vi "Execute.vi"(8 "error in (no error)":errorcluster, 10 "Shifted Error in":refnum<class "Error.lvclass">, 11 "ERROR_Write in":refnum<class "ERROR_Write.lvclass">) -> (0 "error out":errorcluster, 1 "STOP?":bool, 2 "Shifted Error out":refnum<class "Error.lvclass">, 3 "ERROR_Write out":refnum<class "ERROR_Write.lvclass">)   [LabVIEW 2019, in "TSC Error.lvlib" / "ERROR_Write.lvclass"]
doc: "This VI will write the error information to an error log. It contains the following data:\n\nDate String Time String\nVI Name\nMessage: \nGenerated Error Message\n\nInputs:\n-ERROR_Write in [obj] - the dynamic dispatch input class\n-Shifted Error in [obj] - the shifted error class with shared information\n-error in\n\nOutputs:\n-ERROR_Write out [obj] - the dynamic dispatch output class\n-Shifted Error in [obj] - the shifted error class with shared information\n-STOP? [Boolean] - the output Boolean used to stop the Error Loop\n-error out\n\n<b>Code Developed By:</b>\nDaniel Coons\nTechnology Service Corporation\n1983 S Liberty Drive\nBloomington, IN 47403\nPhone: 812 558-7100\nwww.tsc.com/atcs"
uses:
  ERROR_Write.lvclass
  C:/Development/Open Source/tsc-error-library/_Messages/Error/Error.lvclass
  Error/Error.lvclass
  <vilib>/Utility/error.llb/DialogType.ctl
  Error/Error.lvclass/Error.ctl
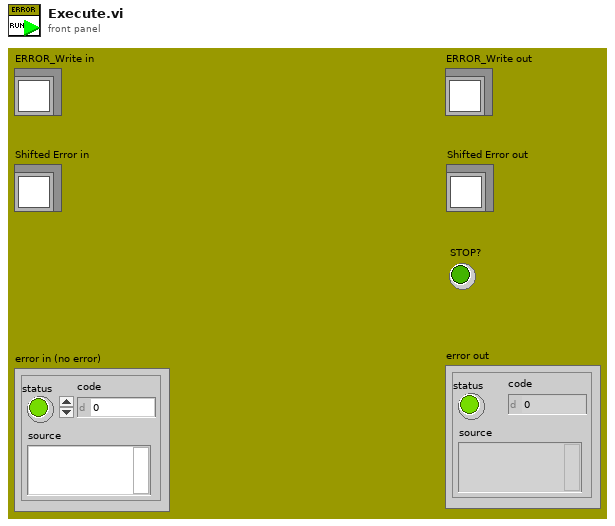
[diagram p1: front panel]
types:
  T1 = typedef "DialogType.ctl" = u16
  T2 = enum16{"open", "replace", "create", "open or create", "replace or create", "replace or create with confirmation"}
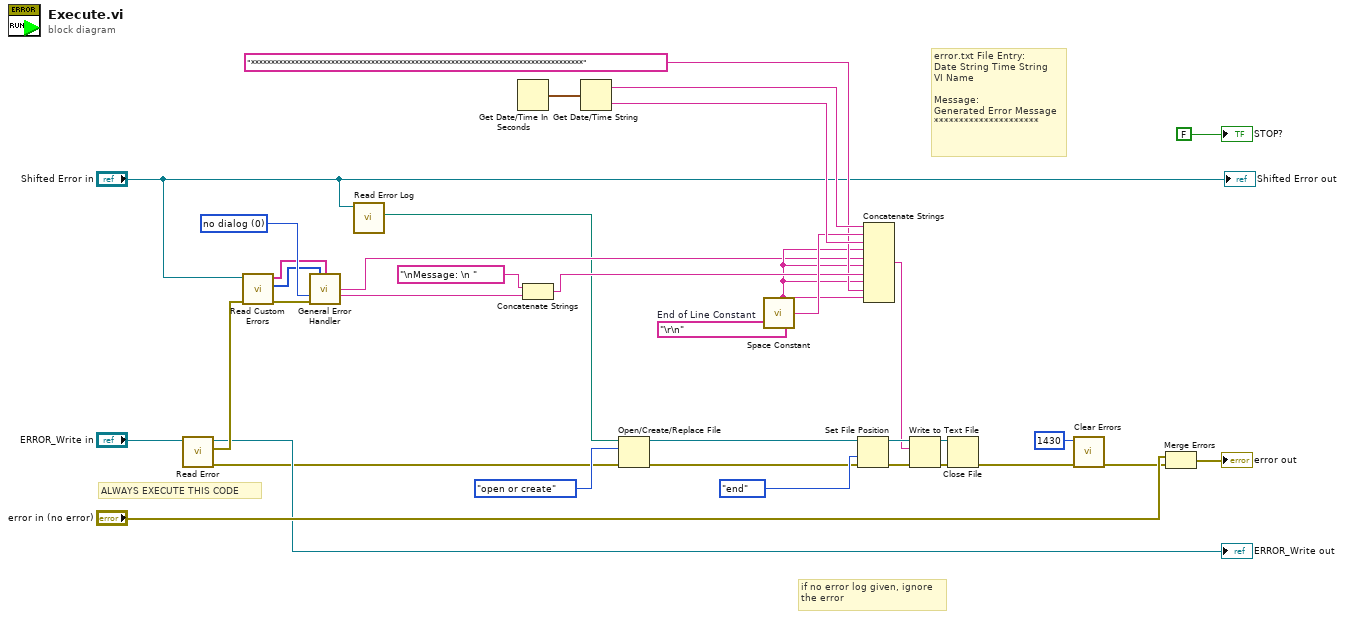
[diagram p0: block diagram]
diagram:
  w18 = T1 0 items=["no dialog", "OK message", "continue or stop message", "OK message + warnings", "continue/stop + warnings"] ("type of dialog (OK msg:1)")
  w13 = "\r\n"  # End of Line Constant
  # "if no error log given, ignore\nthe error"
  # "ALWAYS EXECUTE THIS CODE"
  # "error.txt File Entry:\nDate String Time String\nVI Name\n\nMessage: \nGenerated Error Message\n*********************"
  n1 = call "Read Error.vi"("Error in"="ERROR_Write in") -> ("error out"=w5:errorcluster, "Error"=w11:errorcluster, "Error out"=→"ERROR_Write out":refnum<class "ERROR_Write.lvclass">)  [unwired: 8 in]
  n2 = call "Read Custom Errors.vi"("Error In"=w11, "Error.lvclass"="Shifted Error in") -> ("Error Out"=w10:errorcluster, "Error Codes"=w8:i32[], "Error Messages"=w9:string[])  [unwired: 7 in]
  n3 = call <vilib>:"General Error Handler.vi"("[user-defined codes]"=w8, "[user-defined descriptions]"=w9, "type of dialog (OK msg:1)"=w18, "error in (no error)"=w10) -> ("source out"=w7:string, "message"=w12:string)  [unwired: 7 in, 3 out]
  n4 = call "Read Error Log.vi"("Error in"="Shifted Error in") -> ("Error Log"=w3:path)  [unwired: 8 in, 2 out]
  n5 = Get Date/Time In Seconds() -> (seconds since 1Jan1904=w23:timestamp)
  n6 = Concatenate Strings("\nMessage: \n " ("string"), w12) -> (w15:string)
  n7 = Get Date/Time String(seconds (now)=w23) -> (date string=w22:string, time string=w21:string)  [unwired: 2 in]
  n8 = Open/Create/Replace File(file path (use dialog)=w3, error in=w5, operation (0:open)=T2."open or create") -> (refnum out=w31:refnum<file>, error out=w28:errorcluster)  [unwired: 3 in, 1 out]
  n9 = call <vilib>:"Space Constant.vi"() -> ("String"=w17:string)
  n10 = Set File Position(refnum=w31, from (0:start)=enum16{"start", "end", "current"}."end", error in=w28) -> (refnum out=w30:refnum<file>, error out=w27:errorcluster)  [unwired: 1 in]
  n11 = Concatenate Strings(w22, w17, w21, w13, w7, w13, w15, w13, "***********************************************************************************", w13) -> (w19:string)
  n12 = Write to Text File(file (use dialog)=w30, text=w19, error in=w27) -> (refnum out=w25:refnum<file>, error out=w26:errorcluster)  [unwired: 1 in, 1 out]
  n13 = Close File(refnum=w25, error in=w26) -> (error out=w20:errorcluster)  [unwired: 1 out]
  n14 = call <vilib>:"Clear Errors.vi"("error in (no error)"=w20, "specific error code to clear (0: all)"=1430 ("Error Code")) -> ("error out"=w2:errorcluster)  [unwired: 4 in, 1 out]
  n15 = Merge Errors("error in (no error)", w2) -> (→"error out":errorcluster)
  "STOP?" <- FALSE ("STOP?")
  "Shifted Error out" <- "Shifted Error in"
